vi "Initialize Inset.vi"(8 "error in":errorcluster, 9 "Other Images":refnum<class "SVGImage.lvclass">[](array[class]), 10 "Background Image":refnum<class "SVGImage.lvclass">, 11 "Paths":T1) -> (0 "error out":errorcluster, 3 "Inset out":refnum<class "Inset.lvclass">)   [LabVIEW 2019, in "Inset.lvclass"]
uses:
  Inset.lvclass
  Parse/Image/SVGImage.lvclass
  Inset.lvclass/Inset.ctl
panel:
  in  "Inset in":refnum<class "Inset.lvclass">
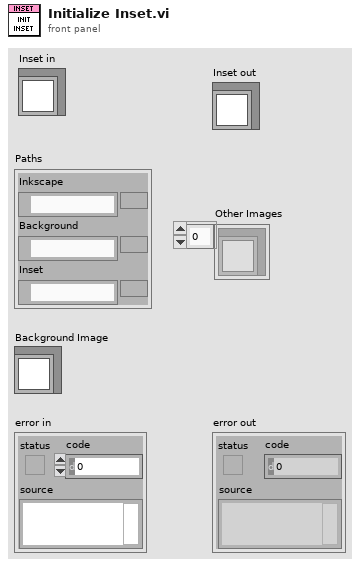
[diagram p1: front panel]
types:
  T1 = cluster{"Inkscape":path, "Background":path, "Inset":path}
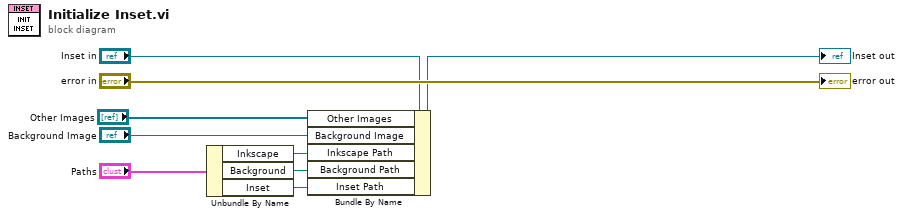
[diagram p0: block diagram]
diagram:
  n1 = Unbundle By Name("Paths") -> ("Inkscape"=w5:path, "Background"=w4:path, "Inset"=w3:path)
  n2 = Bundle By Name(cluster="Inset in", "Other Images"="Other Images", "Background Image"="Background Image", "Inkscape Path"=w5, "Background Path"=w4, "Inset Path"=w3) -> (→"Inset out":refnum<class "Inset.lvclass">)
  "error out" <- "error in"
